vi "Extract data for graph.vi"(8 "error in (no error)":errorcluster, 11 "Data In":T3) -> (0 "error out":errorcluster, 1 "Formatted data for TimeLine graph":T1, 3 "Formatted data for main graph":T1, 4 "Number of points in Timeline graph":i32, 5 "Number of points in main graph":i32)   [LabVIEW 2013, in "XGrapher.xctl"]
uses:
  XGrapher.xctl
  Data 1.ctl
  Typedefs/Xctrl-Data array.ctl
  Typedefs/Xcrtl-Data format definition.ctl
  Typedefs/Xctl-XY data type definition.ctl
  Typedefs/Xctrl-ROI type enum.ctl
  Typedefs/Xctrl-XY Graph data type definition.ctl
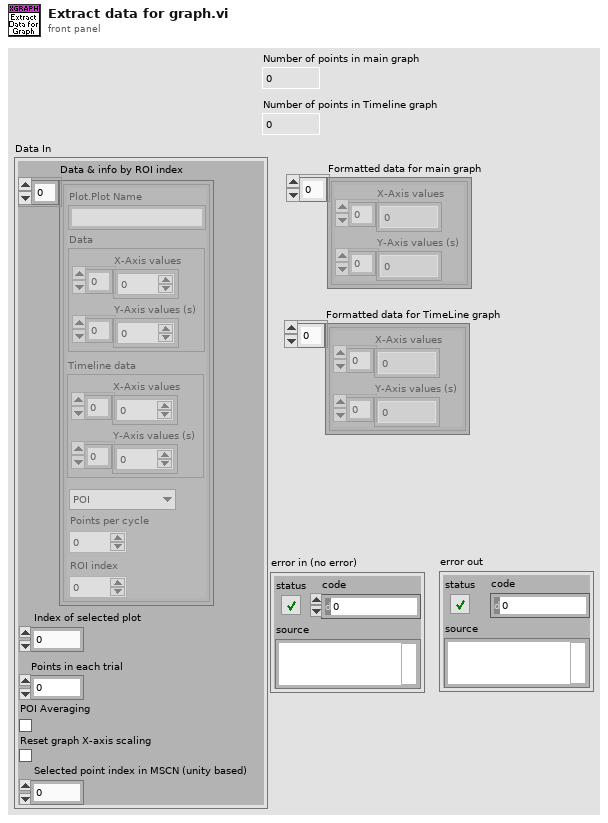
[diagram p1: front panel]
types:
  T1 = typedef "XGrapher.xctl/Xctrl-XY Graph data type definition.ctl" = T2[]
  T2 = typedef "XGrapher.xctl/Xctl-XY data type definition.ctl" = cluster{"X-Axis values":sgl[], "Y-Axis values (s)":i32[]}
  T3 = typedef "XGrapher.xctl/Data 1.ctl" = cluster{"Data & info by ROI index":T4, "Index of selected plot":u16, "Points in each trial":i32, "POI Averaging":bool, "Reset graph X-axis scaling":bool, "Selected point index in MSCN (unity based)":u16}
  T4 = typedef "Xctrl-Data array.ctl" = T5[]
  T5 = typedef "XGrapher.xctl/Xcrtl-Data format definition.ctl" = cluster{"Plot.Plot Name":string, "Data":T2, "Timeline data":T2, "Type":T6, "Points per cycle":u16, "ROI index":u16}
  T6 = typedef "Xctrl-ROI type enum.ctl" = enum16{"POI", "Mini-scan", "Group"}
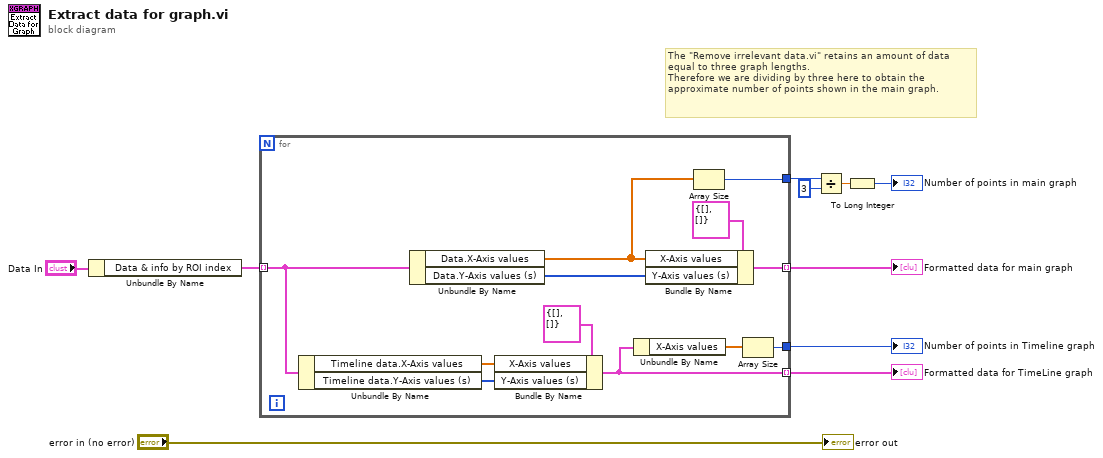
[diagram p0: block diagram]
diagram:
  # "The \"Remove irrelevant data.vi\" retains an amount of data equal to three graph lengths.\nTherefore we are dividing by three here to obtain the approximate number of points shown in the main graph."
  n1 = Unbundle By Name("Data In") -> ("Data & info by ROI index"=w6:T4)
  n2 = for {
    tunnel: w6 -> [w16] mode=indexing
    tunnel: [w21] -> w9 mode=indexing
    tunnel: [w19] -> w8 mode=indexing
    tunnel: [w20] -> w3
    tunnel: [w17] -> w7
    n3 = Unbundle By Name(w16) -> ("Timeline data.X-Axis values"=w14:sgl[], "Timeline data.Y-Axis values (s)"=w13:i32[])
    n4 = Unbundle By Name(w16) -> ("Data.X-Axis values"=w11:sgl[], "Data.Y-Axis values (s)"=w12:i32[])
    n5 = Bundle By Name(cluster=T2 {"X-Axis values"=[], "Y-Axis values (s)"=[]} ("Data 2"), "X-Axis values"=w14, "Y-Axis values (s)"=w13) -> (w19:T2)
    n6 = Unbundle By Name(w19) -> ("X-Axis values"=w18:sgl[])
    n7 = Bundle By Name(cluster=T2 {"X-Axis values"=[], "Y-Axis values (s)"=[]} ("ROI XY waveform data"), "X-Axis values"=w11, "Y-Axis values (s)"=w12) -> (w21:T2)
    n8 = Array Size(array=w11) -> (size(s)=w20:i32)
    n9 = Array Size(array=w18) -> (size(s)=w17:i32)
  }
  "Formatted data for main graph" <- w9
  "Formatted data for TimeLine graph" <- w8
  "Number of points in Timeline graph" <- w7
  n10 = Divide(x=w3, y=3) -> (x/y=w4:dbl)
  n11 = To Long Integer(number=w4) -> (32bit integer=→"Number of points in main graph":i32)
  "error out" <- "error in (no error)"
